vi "translational.vi"() -> ()   [LabVIEW 2019]
uses:
  <vilib>/MakerHub/LINX/Public/Utilities/Open Serial.vi
  <vilib>/picture/3D Picture Control/Object/Create Object (drawable).vi
  <vilib>/ErrorRing/Error Ring.xnode
  <vilib>/MakerHub/LINX/Public/Sensors/Accelerometer/ADXL345/ADXL345.lvlib
  <vilib>/MakerHub/LINX/LMH-LINX.lvlib
  <vilib>/picture/3D Picture Control/NI_3D Picture Control.lvlib
panel:
  in  "Color 2":T1={"Red"=1.0, "Green"=0.0, "Blue"=0.0, "Alpha"=1.0}
  out "3D Picture":refnum<vi>(3d-picture)
  out "Waveform Chart":T2(graph)
  in  "I2C Channel (0)":u8
  in  "Serial Port":refnum<visa-resource-name>="N/A"
  in  "stop":bool
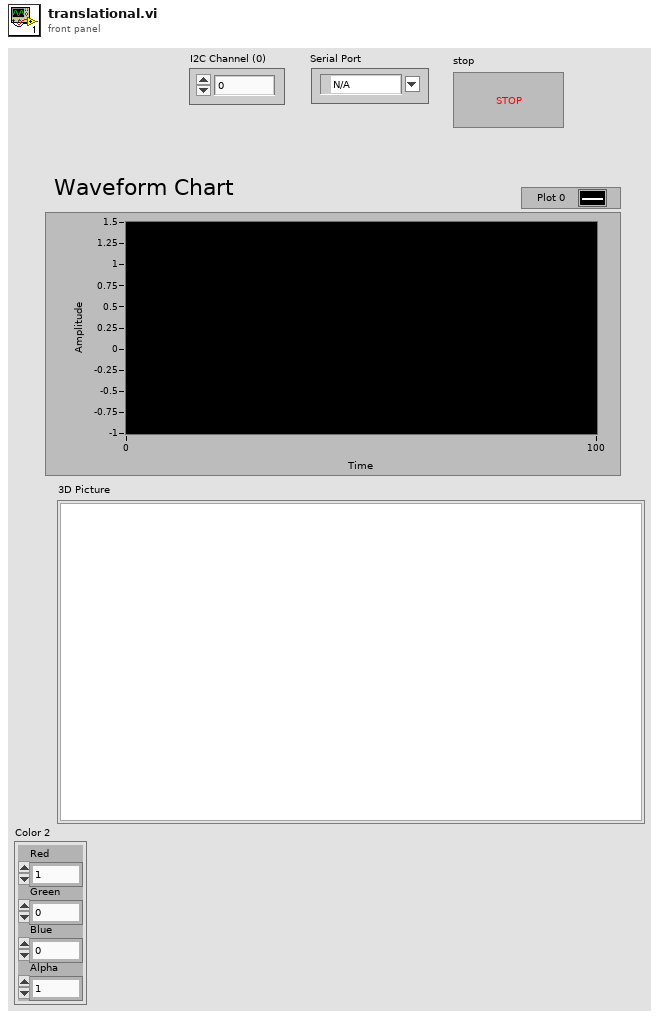
[diagram p1: front panel]
types:
  T1 = cluster{"Red":sgl, "Green":sgl, "Blue":sgl, "Alpha":sgl}
  T2 = cluster{"X Axis":dbl, "Y Axis":dbl, "Z Axis":dbl}
  T3 = typedef "LMH-LINX.lvlib/LINX Ref.ctl" = cluster{"IO":T4, "Interface":T5, "LINX Device Config":T6}
  T4 = typedef "LMH-LINX.lvlib/Platform.ctl" = enum16{"Remote", "Local"}
  T5 = typedef "LMH-LINX.lvlib/Interface.ctl" = enum16{"Serial", "TCP"}
  T6 = typedef "LMH-LINX.lvlib/Device.lvlib/LINX Device Config.ctl" = cluster{"Interface":T5, "COM Port":refnum<visa-resource-name>, "TCP Configuration":T7, "Device Family":u8, "Device ID":u8, "Device Name":string, "TCP Ref":refnum<k5>, "Channels":T8}
  T7 = typedef "LMH-LINX.lvlib/Device.lvlib/TCP Config.ctl" = cluster{"IP Address":string, "Port":u16}
  T8 = typedef "LMH-LINX.lvlib/Channels.ctl" = cluster{"DI":u8[], "DO":u8[], "AI":u8[], "AO":u8[], "PWM":u8[], "QE":u8[], "UART":u8[], "I2C 2":u8[], "SPI":u8[], "CAN":u8[], "Servo":u8[], "AI Ref (V)":dbl, "AI Resolution (Bits)":u8, "AO Ref (V)":dbl, "AO Resolution (Bits)":u8}
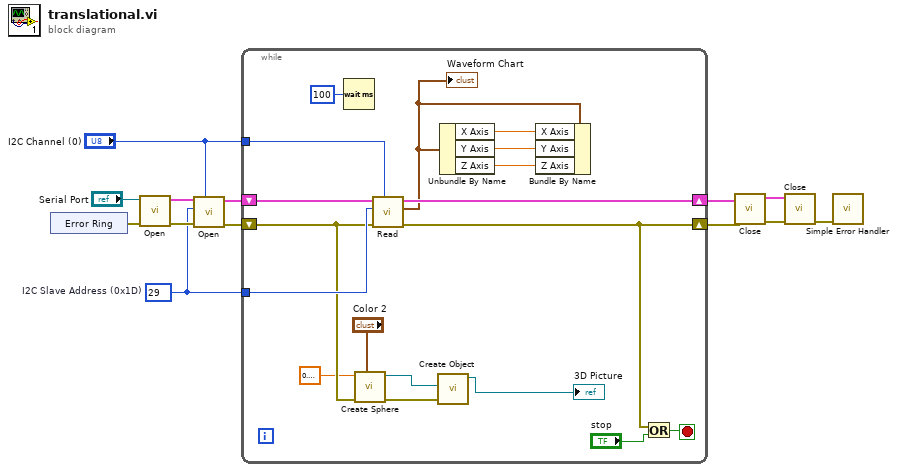
[diagram p0: block diagram]
diagram:
  w1 = u8 29  # I2C Slave Address (0x1D)
  n1 = xnode "Error Ring"() -> ("error out"=w3:errorcluster)
  n2 = call-poly <vilib>:"Open.vi"("Error In"=w3, "Serial Port"="Serial Port") -> ("Error Out"=w7:errorcluster, "LINX Resource"=w10:T3)  [unwired: 7 in, 1 out]
  n3 = call <vilib>:"Open.vi"("I2C Channel (0)"="I2C Channel (0)", "Error In"=w7, "I2C Slave Address"=w1, "LINX Resource"=w10) -> ("Error Out"=w6:errorcluster, "LINX Resource"=w9:T3)  [unwired: 5 in, 1 out]
  n4 = while {
    tunnel: "I2C Channel (0)" -> [w26]
    tunnel: w1 -> [w25]
    shift-right: [w30] -> w8
    shift-left: w9 -> [w31]
    shift-right: [w27] -> w5
    shift-left: w6 -> [w19]
    stop <- w29 stop-if-true
    n5 = Wait (ms)(milliseconds to wait=u32 100) -> ()  [unwired: 1 out]
    n6 = call <vilib>:"Create Sphere.vi"("Color"="Color 2", "error in (no error)"=w19, "Radius"=sgl 0.2) -> ("error out"=w17:errorcluster, "New Sphere Refnum"=w18:refnum<vi>)  [unwired: 7 in]
    n7 = call <vilib>:"Read.vi"("I2C Channel (0)"=w26, "Error In"=w19, "I2C Slave Address"=w25, "LINX Resource"=w31) -> ("Error Out"=w27:errorcluster, "Acceleration Data (g)"=w22:T2, "LINX Resource"=w30:T3)  [unwired: 5 in]
    "Waveform Chart" <- w22
    n8 = call-poly <vilib>:"Create Object.vi"("error in (no error)"=w17, "Geometry"=w18) -> ("Scene:New Object"=→"3D Picture":refnum<vi>)  [unwired: 8 in, 1 out]
    n9 = Unbundle By Name(w22) -> ("X Axis"=w21:dbl, "Y Axis"=w20:dbl, "Z Axis"=w23:dbl)
    n10 = Bundle By Name(cluster=w22, "X Axis"=w21, "Y Axis"=w20, "Z Axis"=w23) -> ()  [unwired: 1 out]
    n11 = Or(x=w27, y="stop") -> (x .or. y?=w29:bool)
  }
  n12 = call <vilib>:"Close.vi"("Error In"=w5, "LINX Resource"=w8) -> ("Error Out"=w13:errorcluster, "LINX Resource"=w12:T3)  [unwired: 8 in]
  n13 = call <vilib>:"Close.vi"("Error In"=w13, "LINX Resource"=w12) -> ("Error Out"=w11:errorcluster)  [unwired: 9 in]
  n14 = call <vilib>:"Simple Error Handler.vi"("error in (no error)"=w11) -> ()  [unwired: 4 in, 5 out]
